vi "ethernet_ip_Test Panel.vi"(8 "Error In":errorcluster) -> (0 "Error Out":errorcluster)   [LabVIEW 2020]
doc: "Use this template to build a producer/consumer design pattern with events to produce queue items. Use this design pattern instead of the User Interface Event Handler pattern for user interfaces when you want to execute code asynchronously in response to an event without slowing the user interface responsiveness."
uses:
  EIP.ctl
panel:
  out "size(s)":i32
  in  "STRING in":string
  in  "RAW U8 in":u8[](array[numeric])
  in  "BOOL in":bool[](array[boolean])
  in  "SGL in":sgl[](array[numeric])
  in  "32INT in":i32[](array[numeric])
  in  "16INT in":i16[](array[numeric])
  in  "8INT in":i8[](array[numeric])
  in  "Tag Name":string
  in  "Number of Elements":u32=1
  out "RAW U8 out":u8[](array[numeric])
  out "BOOL out":bool[](array[boolean])
  out "STRING out":string
  out "SGL out":sgl[](array[numeric])
  out "32INT out":i32[](array[numeric])
  out "16INT out":i16[](array[numeric])
  out "8INT out":i8[](array[numeric])
  in  "EIP":T1
  in  "Enqueue Element":bool
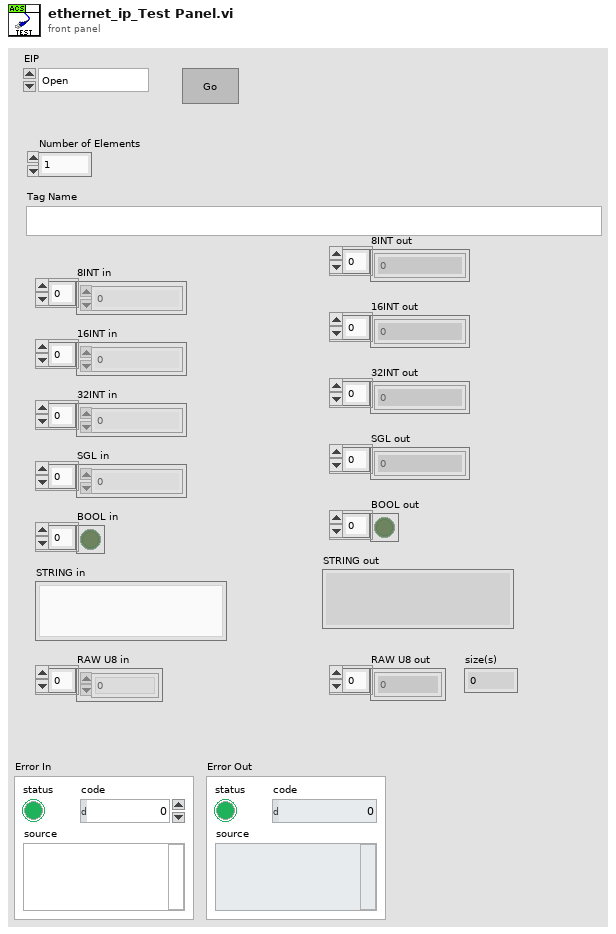
[diagram p1: front panel]
types:
  T1 = typedef "EIP.ctl" = enum16{"Open", "Close", "Tag Read SINT", "Tag Read INT", "Tag Read DINT", "Tag Read REAL", "Tag Read BOOL", "Tag Read STRING", "Tag Read RAW", "Tag Write SINT", "Tag Write INT", "Tag Write DINT", "Tag Write REAL", "Tag Write BOOL", "Tag Write STRING", "Tag Write Raw"}
  T2 = typedef "ethernetip.lvlib/ethernetip.ctl" = refnum<k21>
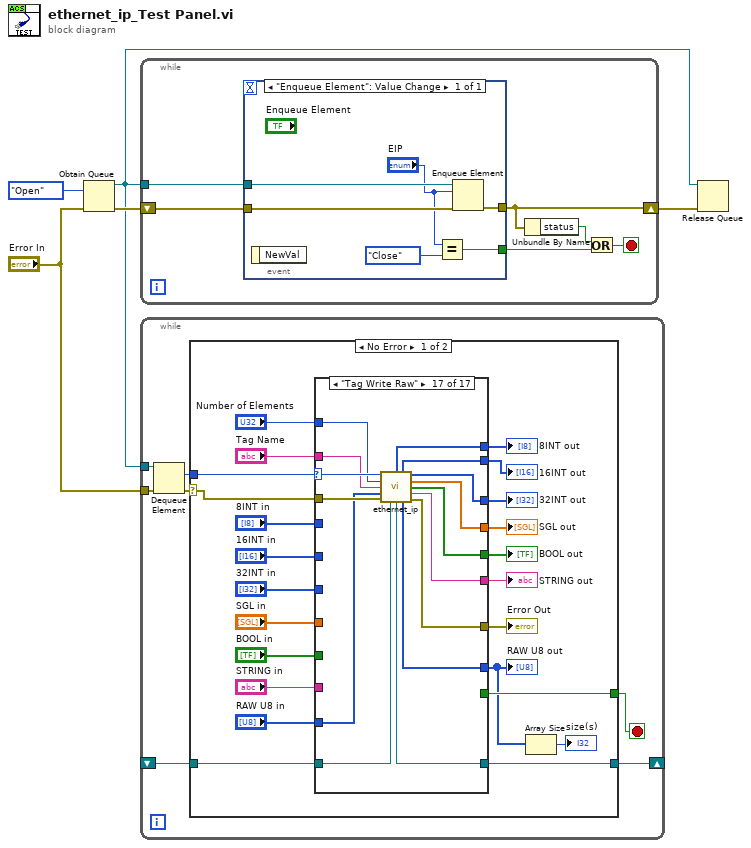
[diagram p0: block diagram]
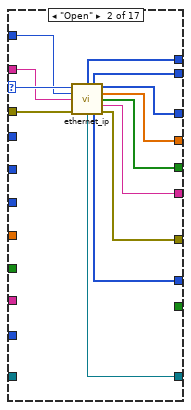
[diagram p3: hidden frame]
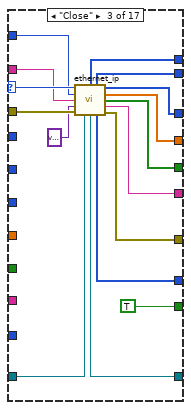
[diagram p4: hidden frame]
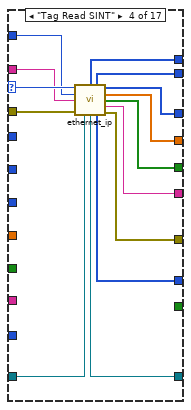
[diagram p5: hidden frame]
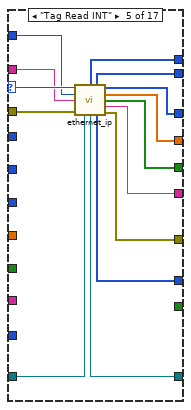
[diagram p6: hidden frame]
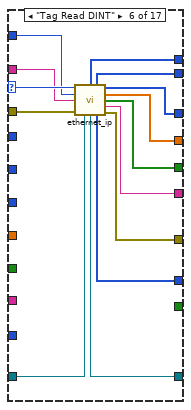
[diagram p7: hidden frame]
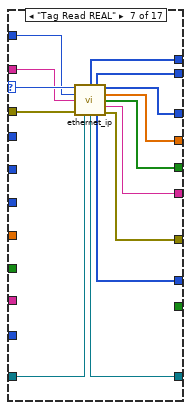
[diagram p8: hidden frame]
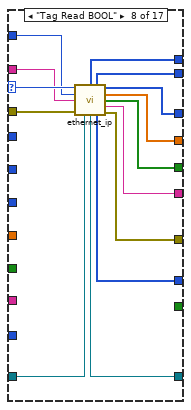
[diagram p9: hidden frame]
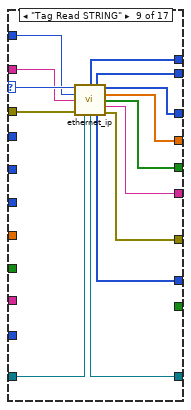
[diagram p10: hidden frame]
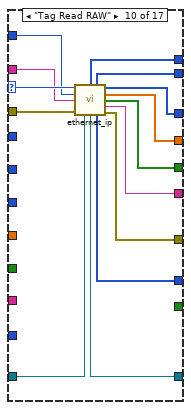
[diagram p11: hidden frame]
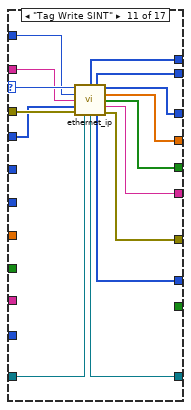
[diagram p12: hidden frame]
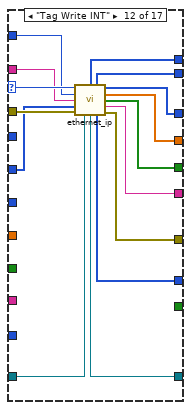
[diagram p13: hidden frame]
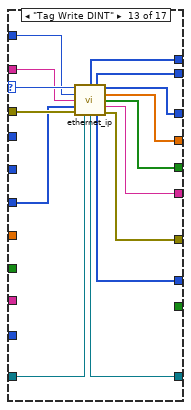
[diagram p14: hidden frame]
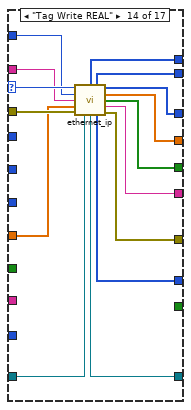
[diagram p15: hidden frame]
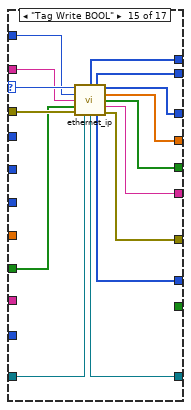
[diagram p16: hidden frame]
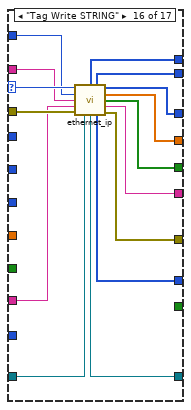
[diagram p17: hidden frame]
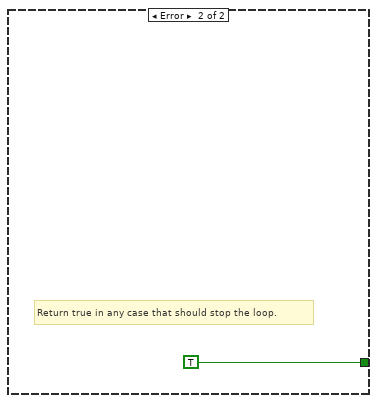
[diagram p18: hidden frame]
diagram:
  n1 = Obtain Queue(element data type=EIP."Open" ("EIP"), error in (no error)="Error In") -> (queue out=w3:refnum<queue>, error out=w5:errorcluster)  [unwired: 3 in, 1 out]
  n2 = while {
    shift-right: [w7] -> w4
    shift-left: w5 -> [w10]
    tunnel: w3 -> [w11]
    stop <- w8 stop-if-true
    n3 = event shown="[0] \"Enqueue Element\": Value Change" {
      selector: _ -> [_]
      dyn-events: _ -> [_]
      timeout: _ -> [_]
      tunnel: w11 -> [w17]
      tunnel: w10 -> [w16]
      tunnel: [w15] -> w7
      tunnel: [w12] -> w9
      event "Enqueue Element": Value Change {
        n4 = event-data() -> ()  [unwired: 1 in, 1 out]
        n5 = Equal?(x="EIP", y=EIP."Close" ("EIP")) -> (x = y?=w12:bool)
        n6 = Enqueue Element(queue=w17, element="EIP", error in (no error)=w16) -> (error out=w15:errorcluster)  [unwired: 1 in, 2 out]
      }
    }
    n7 = Unbundle By Name(w7) -> ("status"=w6:bool)
    n8 = Or(x=w6, y=w9) -> (x .or. y?=w8:bool)
  }
  n9 = while {
    tunnel: w3 -> [w24]
    tunnel: "Error In" -> [w20]
    shift-right: [w19] -> _
    shift-left: _ -> [w18]
    stop <- w21 stop-if-true
    n10 = Dequeue Element(queue=w24, error in (no error)=w20) -> (element=w22:T1, error out=w23:errorcluster)  [unwired: 1 in, 2 out]
    n11 = case shown="No Error" w23 {
      selector: w23 -> [w46 _]
      tunnel: w22 -> [w47 _]
      tunnel: [w29 TRUE] -> w21
      tunnel: [w26 _] -> w19
      tunnel: w18 -> [w25 _]
      frame No Error {
        n12 = case shown="\"Tag Write Raw\"" w47 {
          selector: w47 -> [_ w61 w77 w91 w105 w119 w133 w147 w161 w175 w190 w205 w220 w235 w250 w265 w280]
          tunnel: w46 -> [_ w60 w76 w90 w104 w118 w132 w146 w160 w174 w189 w204 w219 w234 w249 w264 w279]
          tunnel: [_ w59 w75 w89 w103 w117 w131 w145 w159 w173 w188 w203 w218 w233 w248 w263 w278] -> w45
          tunnel: "Tag Name" -> [_ w51 w66 w88 w102 w116 w130 w144 w158 w172 w187 w202 w217 w232 w247 w262 w277]
          tunnel: "Number of Elements" -> [_ w50 w67 w87 w101 w115 w129 w143 w157 w171 w186 w201 w216 w231 w246 w261 w276]
          tunnel: [_ w58 w74 w86 w99 w113 w126 w141 w155 w169 w184 w199 w214 w229 w244 w259 w274] -> w42
          tunnel: [_ w57 w73 w85 w100 w112 w125 w140 w154 w168 w183 w198 w213 w228 w243 w258 w273] -> w41
          tunnel: [_ w56 w72 w84 w98 w114 w124 w139 w153 w167 w182 w197 w212 w227 w242 w257 w272] -> w40
          tunnel: [_ w55 w71 w83 w97 w111 w128 w138 w152 w166 w181 w196 w211 w226 w241 w256 w271] -> w39
          tunnel: [_ w54 w70 w82 w96 w110 w123 w142 w151 w165 w180 w195 w210 w225 w240 w255 w270] -> w38
          tunnel: [_ w53 w69 w81 w95 w109 w122 w136 w156 w170 w185 w200 w215 w230 w245 w260 w275] -> w37
          tunnel: [_ w52 w68 w80 w94 w108 w127 w137 w150 w164 w179 w194 w209 w224 w239 w254 w269] -> w28
          tunnel: "8INT in" -> [_ _ _ _ _ _ _ _ _ _ w178 _ _ _ _ _ _]
          tunnel: "16INT in" -> [_ _ _ _ _ _ _ _ _ _ _ w193 _ _ _ _ _]
          tunnel: "32INT in" -> [_ _ _ _ _ _ _ _ _ _ _ _ w208 _ _ _ _]
          tunnel: "SGL in" -> [_ _ _ _ _ _ _ _ _ _ _ _ _ w223 _ _ _]
          tunnel: "BOOL in" -> [_ _ _ _ _ _ _ _ _ _ _ _ _ _ w238 _ _]
          tunnel: "STRING in" -> [_ _ _ _ _ _ _ _ _ _ _ _ _ _ _ w253 _]
          tunnel: "RAW U8 in" -> [_ _ _ _ _ _ _ _ _ _ _ _ _ _ _ _ w268]
          tunnel: [_ _ TRUE _ _ _ _ _ _ _ _ _ _ _ _ _ _] -> w29
          tunnel: [w48 w49 w62 w78 w92 w106 w120 w134 w148 w162 w176 w191 w206 w221 w236 w251 w266] -> w26
          tunnel: w25 -> [w48 _ w63 w79 w93 w107 w121 w135 w149 w163 w177 w192 w207 w222 w237 w252 w267]
          frame Default {
          }
          frame "Open" {
            n13 = call "ethernet_ip.vi"("EIP"=w61, "Number of Elements"=w50, "Tag Name"=w51, "error in (no error)"=w60) -> ("8INT out"=w58:i8[], "16INT out"=w57:i16[], "32INT out"=w56:i32[], "SGL out"=w55:sgl[], "BOOL out"=w54:bool[], "STRING out"=w53:string, "Session out"=w49:T2, "RAW U8 out"=w52:u8[], "error out"=w59:errorcluster)  [unwired: 3 in]
          }
          frame "Close" {
            n14 = call "ethernet_ip.vi"("EIP"=w77, "Number of Elements"=w67, "Tag Name"=w66, "data in"=variant, "error in (no error)"=w76, "Session in"=w63) -> ("8INT out"=w74:i8[], "16INT out"=w73:i16[], "32INT out"=w72:i32[], "SGL out"=w71:sgl[], "BOOL out"=w70:bool[], "STRING out"=w69:string, "Session out"=w62:T2, "RAW U8 out"=w68:u8[], "error out"=w75:errorcluster)  [unwired: 1 in]
          }
          frame "Tag Read SINT" {
            n15 = call "ethernet_ip.vi"("EIP"=w91, "Number of Elements"=w87, "Tag Name"=w88, "error in (no error)"=w90, "Session in"=w79) -> ("8INT out"=w86:i8[], "16INT out"=w85:i16[], "32INT out"=w84:i32[], "SGL out"=w83:sgl[], "BOOL out"=w82:bool[], "STRING out"=w81:string, "Session out"=w78:T2, "RAW U8 out"=w80:u8[], "error out"=w89:errorcluster)  [unwired: 2 in]
          }
          frame "Tag Read INT" {
            n16 = call "ethernet_ip.vi"("EIP"=w105, "Number of Elements"=w101, "Tag Name"=w102, "error in (no error)"=w104, "Session in"=w93) -> ("8INT out"=w99:i8[], "16INT out"=w100:i16[], "32INT out"=w98:i32[], "SGL out"=w97:sgl[], "BOOL out"=w96:bool[], "STRING out"=w95:string, "Session out"=w92:T2, "RAW U8 out"=w94:u8[], "error out"=w103:errorcluster)  [unwired: 2 in]
          }
          frame "Tag Read DINT" {
            n17 = call "ethernet_ip.vi"("EIP"=w119, "Number of Elements"=w115, "Tag Name"=w116, "error in (no error)"=w118, "Session in"=w107) -> ("8INT out"=w113:i8[], "16INT out"=w112:i16[], "32INT out"=w114:i32[], "SGL out"=w111:sgl[], "BOOL out"=w110:bool[], "STRING out"=w109:string, "Session out"=w106:T2, "RAW U8 out"=w108:u8[], "error out"=w117:errorcluster)  [unwired: 2 in]
          }
          frame "Tag Read REAL" {
            n18 = call "ethernet_ip.vi"("EIP"=w133, "Number of Elements"=w129, "Tag Name"=w130, "error in (no error)"=w132, "Session in"=w121) -> ("8INT out"=w126:i8[], "16INT out"=w125:i16[], "32INT out"=w124:i32[], "SGL out"=w128:sgl[], "BOOL out"=w123:bool[], "STRING out"=w122:string, "Session out"=w120:T2, "RAW U8 out"=w127:u8[], "error out"=w131:errorcluster)  [unwired: 2 in]
          }
          frame "Tag Read BOOL" {
            n19 = call "ethernet_ip.vi"("EIP"=w147, "Number of Elements"=w143, "Tag Name"=w144, "error in (no error)"=w146, "Session in"=w135) -> ("8INT out"=w141:i8[], "16INT out"=w140:i16[], "32INT out"=w139:i32[], "SGL out"=w138:sgl[], "BOOL out"=w142:bool[], "STRING out"=w136:string, "Session out"=w134:T2, "RAW U8 out"=w137:u8[], "error out"=w145:errorcluster)  [unwired: 2 in]
          }
          frame "Tag Read STRING" {
            n20 = call "ethernet_ip.vi"("EIP"=w161, "Number of Elements"=w157, "Tag Name"=w158, "error in (no error)"=w160, "Session in"=w149) -> ("8INT out"=w155:i8[], "16INT out"=w154:i16[], "32INT out"=w153:i32[], "SGL out"=w152:sgl[], "BOOL out"=w151:bool[], "STRING out"=w156:string, "Session out"=w148:T2, "RAW U8 out"=w150:u8[], "error out"=w159:errorcluster)  [unwired: 2 in]
          }
          frame "Tag Read RAW" {
            n21 = call "ethernet_ip.vi"("EIP"=w175, "Number of Elements"=w171, "Tag Name"=w172, "error in (no error)"=w174, "Session in"=w163) -> ("8INT out"=w169:i8[], "16INT out"=w168:i16[], "32INT out"=w167:i32[], "SGL out"=w166:sgl[], "BOOL out"=w165:bool[], "STRING out"=w170:string, "Session out"=w162:T2, "RAW U8 out"=w164:u8[], "error out"=w173:errorcluster)  [unwired: 2 in]
          }
          frame "Tag Write SINT" {
            n22 = call "ethernet_ip.vi"("EIP"=w190, "Number of Elements"=w186, "Tag Name"=w187, "data in"=w178, "error in (no error)"=w189, "Session in"=w177) -> ("8INT out"=w184:i8[], "16INT out"=w183:i16[], "32INT out"=w182:i32[], "SGL out"=w181:sgl[], "BOOL out"=w180:bool[], "STRING out"=w185:string, "Session out"=w176:T2, "RAW U8 out"=w179:u8[], "error out"=w188:errorcluster)  [unwired: 1 in]
          }
          frame "Tag Write INT" {
            n23 = call "ethernet_ip.vi"("EIP"=w205, "Number of Elements"=w201, "Tag Name"=w202, "data in"=w193, "error in (no error)"=w204, "Session in"=w192) -> ("8INT out"=w199:i8[], "16INT out"=w198:i16[], "32INT out"=w197:i32[], "SGL out"=w196:sgl[], "BOOL out"=w195:bool[], "STRING out"=w200:string, "Session out"=w191:T2, "RAW U8 out"=w194:u8[], "error out"=w203:errorcluster)  [unwired: 1 in]
          }
          frame "Tag Write DINT" {
            n24 = call "ethernet_ip.vi"("EIP"=w220, "Number of Elements"=w216, "Tag Name"=w217, "data in"=w208, "error in (no error)"=w219, "Session in"=w207) -> ("8INT out"=w214:i8[], "16INT out"=w213:i16[], "32INT out"=w212:i32[], "SGL out"=w211:sgl[], "BOOL out"=w210:bool[], "STRING out"=w215:string, "Session out"=w206:T2, "RAW U8 out"=w209:u8[], "error out"=w218:errorcluster)  [unwired: 1 in]
          }
          frame "Tag Write REAL" {
            n25 = call "ethernet_ip.vi"("EIP"=w235, "Number of Elements"=w231, "Tag Name"=w232, "data in"=w223, "error in (no error)"=w234, "Session in"=w222) -> ("8INT out"=w229:i8[], "16INT out"=w228:i16[], "32INT out"=w227:i32[], "SGL out"=w226:sgl[], "BOOL out"=w225:bool[], "STRING out"=w230:string, "Session out"=w221:T2, "RAW U8 out"=w224:u8[], "error out"=w233:errorcluster)  [unwired: 1 in]
          }
          frame "Tag Write BOOL" {
            n26 = call "ethernet_ip.vi"("EIP"=w250, "Number of Elements"=w246, "Tag Name"=w247, "data in"=w238, "error in (no error)"=w249, "Session in"=w237) -> ("8INT out"=w244:i8[], "16INT out"=w243:i16[], "32INT out"=w242:i32[], "SGL out"=w241:sgl[], "BOOL out"=w240:bool[], "STRING out"=w245:string, "Session out"=w236:T2, "RAW U8 out"=w239:u8[], "error out"=w248:errorcluster)  [unwired: 1 in]
          }
          frame "Tag Write STRING" {
            n27 = call "ethernet_ip.vi"("EIP"=w265, "Number of Elements"=w261, "Tag Name"=w262, "data in"=w253, "error in (no error)"=w264, "Session in"=w252) -> ("8INT out"=w259:i8[], "16INT out"=w258:i16[], "32INT out"=w257:i32[], "SGL out"=w256:sgl[], "BOOL out"=w255:bool[], "STRING out"=w260:string, "Session out"=w251:T2, "RAW U8 out"=w254:u8[], "error out"=w263:errorcluster)  [unwired: 1 in]
          }
          frame "Tag Write Raw" {
            n28 = call "ethernet_ip.vi"("EIP"=w280, "Number of Elements"=w276, "Tag Name"=w277, "data in"=w268, "error in (no error)"=w279, "Session in"=w267) -> ("8INT out"=w274:i8[], "16INT out"=w273:i16[], "32INT out"=w272:i32[], "SGL out"=w271:sgl[], "BOOL out"=w270:bool[], "STRING out"=w275:string, "Session out"=w266:T2, "RAW U8 out"=w269:u8[], "error out"=w278:errorcluster)  [unwired: 1 in]
          }
        }
        "Error Out" <- w45
        "STRING out" <- w37
        "BOOL out" <- w38
        "SGL out" <- w39
        "8INT out" <- w42
        "16INT out" <- w41
        "32INT out" <- w40
        "RAW U8 out" <- w28
        n29 = Array Size(array=w28) -> (size(s)=→"size(s)":i32)
      }
      frame Error {
        # "Return true in any case that should stop the loop."
      }
    }
  }
  n30 = Release Queue(queue=w3, error in (no error)=w4) -> ()  [unwired: 1 in, 3 out]
